vi "Get Data.vi"(8 "error in (no error)":errorcluster, 11 "DataGrid.lvlib:Abstract EVENT.lvclass":refnum<class "Abstract EVENT.lvclass">) -> (0 "error out":errorcluster, 2 "Row":refnum<k24>)   [LabVIEW 2014, in "DataGrid.lvlib" / "UserAddedRow.lvclass"]
uses:
  UserAddedRow.lvclass
  Abstract EVENT/Abstract EVENT.lvclass
  System.Windows.Forms
  UserAddedRow.lvclass/UserAddedRow.ctl
  Read Row.vi
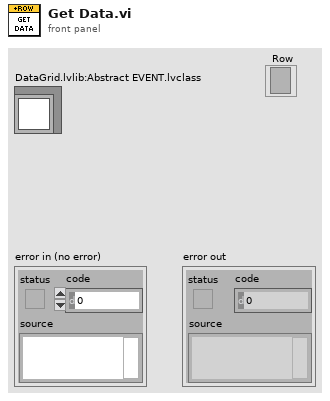
[diagram p1: front panel]
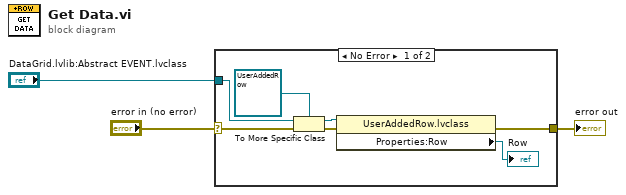
[diagram p0: block diagram]
diagram:
  n1 = case shown="No Error" "error in (no error)" {
    selector: "error in (no error)" -> [w7 w11]
    tunnel: [w10 w11] -> w2
    tunnel: "DataGrid.lvlib:Abstract EVENT.lvclass" -> [w9 _]
    frame No Error {
      n2 = To More Specific Class(target class=refnum<class "UserAddedRow.lvclass"> refnum ("DataGrid.lvlib:UserAddedRow.lvclass"), reference=w9, error in=w7) -> (specific class reference=w8:refnum<class "UserAddedRow.lvclass">, error out=w6:errorcluster)
      n3 = property class="UserAddedRow.lvclass"(reference=w8, error in=w6) -> (error out=w10:errorcluster, "Properties:Row"=→"Row":refnum<k24>)  [unwired: 1 out]
    }
    frame Error {
    }
  }
  "error out" <- w2
